vi "Send Voltage.vi"(8 "error in":errorcluster, 11 "69X_79X in":refnum<class "7976A.lvclass">) -> (0 "error out":errorcluster, 3 "69X_79X out":refnum<class "7976A.lvclass">)   [LabVIEW 2019, in "7976A.lvlib" / "7976A.lvclass"]
uses:
  Library/7976A.lvclass
  C:/Users/Public/Documents/Development/builds/Instruments/PowerSupply.lvlibp/Library/PowerSupply.lvclass
  Library/7976A.lvclass/7976A.ctl
  builds/Engine/Engine.lvlibp/Project/Engine.lvclass
  <instrlib>/Agilent N7976A/Agilent N7976A.lvlib
  C:/Users/Public/Documents/Development/builds/Engine/Engine.lvlibp/Project/Engine.lvclass
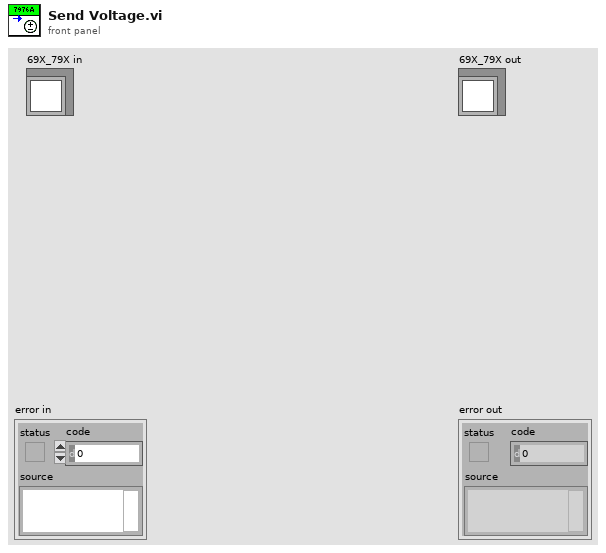
[diagram p1: front panel]
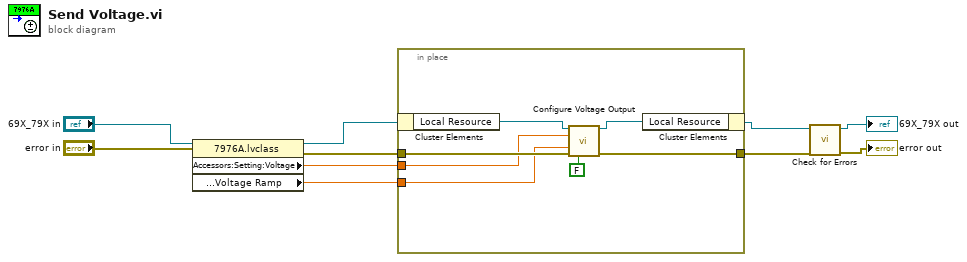
[diagram p0: block diagram]
diagram:
  n1 = property class="7976A.lvclass"(reference="69X_79X in", error in="error in") -> (reference out=w6:refnum<class "7976A.lvclass">, error out=w4:errorcluster, "Accessors:Setting:Voltage"=w2:dbl, "Accessors:Setting:Ramp:Voltage Ramp"=w1:dbl)
  n2 = in-place {
    in-place-border: w4 -> [w15]
    in-place-border: [w14] -> w3
    in-place-border: w2 -> [w13]
    in-place-border: w1 -> [w12]
    n3 = in-place-cluster #1(w6) -> ("Local Resource"=w17:refnum<visa-resource-name>)
    n4 = call <instrlib>:"Configure Voltage Output.vi"("VISA resource name"=w17, "Voltage Immediate Amplitude (0 V)"=w13, "Voltage Slew (Inf)"=w12, "error in (no error)"=w15, "Enable Current Priority (False)"=FALSE) -> ("VISA resource name out"=w16:refnum<visa-resource-name>, "error out"=w14:errorcluster)  [unwired: 9 in]
    n5 = in-place-cluster #1("Local Resource"=w16) -> (w5:refnum<class "7976A.lvclass">)
  }
  n6 = call "Check for Errors.vi"("error in"=w3, "Engine in"=w5) -> ("error out"=→"error out":errorcluster, "Engine out"=→"69X_79X out":refnum<class "7976A.lvclass">)  [unwired: 8 in]
